vi "Destroy.vi"(0 "reference in":refnum<class "NI_DAQ.lvclass">, 5 "error in (no error)":errorcluster) -> (14 "reference out":refnum<class "NI_DAQ.lvclass">, 19 "error out":errorcluster)   [LabVIEW 2020, in "NI_DAQ.lvclass"]
doc: "Destructor."
uses:
  NI_DAQ.lvclass
  DAQ_Base_class/DAQ_Base.lvclass
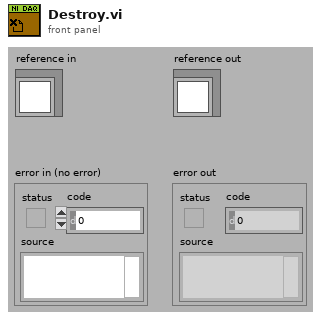
[diagram p1: front panel]
types:
  T1 = typedef "NI_DAQ.lvclass/ObjectAttributes.ctl" = cluster{"MyAttribute":dbl, "DAQ_AI_task_out":refnum<k21>, "counter_task_out":refnum<k21>[]}
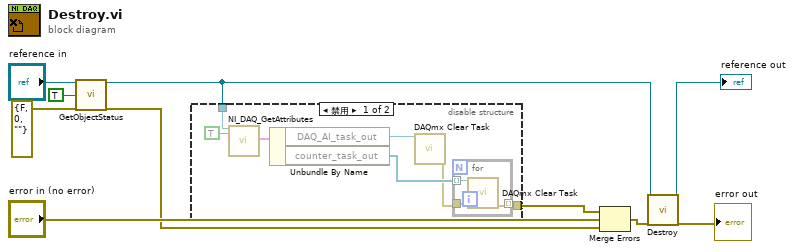
[diagram p0: block diagram]
diagram:
  n1 = call-dynamic "GetObjectStatus.vi"("reference in"="reference in", "simple info (F)"=TRUE ("simple info"), "error in (no error)"=errorcluster {"status"=FALSE, "code"=0, "source"=""}) -> ("reference out"=w2:refnum<class "NI_DAQ.lvclass">, "error out"=w3:errorcluster)  [unwired: 5 in, 10 out]
  n2 = disable-structure shown="禁用" {
    disable-tunnel: w2 -> [w17 _]
    disable-tunnel: [w11 _] -> w1
    frame Disabled {
      n3 = call "NI_DAQ_GetAttributes.vi"("reference in"=w17, "return data? (T)"=TRUE) -> ("attributes"=w15:T1)  [unwired: 14 in, 3 out]
      n4 = Unbundle By Name(w15) -> ("DAQ_AI_task_out"=w14:refnum<k21>, "counter_task_out"=w13:refnum<k21>[])
      n5 = call <vilib>:"DAQmx Clear Task.vi"("task in"=w14) -> ("error out"=w12:errorcluster)  [unwired: 14 in]
      n6 = for {
        tunnel: w13 -> [w20] mode=indexing
        tunnel: w12 -> [w19]
        tunnel: [w18] -> w11 mode=indexing
        n7 = call <vilib>:"DAQmx Clear Task.vi"("task in"=w20, "error in"=w19) -> ("error out"=w18:errorcluster)  [unwired: 13 in]
      }
    }
    frame Enabled {
    }
  }
  n8 = Merge Errors(w1, "error in (no error)", w3) -> (w9:errorcluster)
  n9 = call-parent "Destroy.vi"("reference in"=w2, "error in (no error)"=w9) -> ("reference out"=→"reference out":refnum<class "NI_DAQ.lvclass">, "error out"=→"error out":errorcluster)  [unwired: 16 in]
